vi "SetExposure.vi"(8 "error in (no error)":errorcluster, 10 "Exposure":dbl, 11 "CameraSession  in":refnum<class "CS250-CameraHardwareClass.lvclass">) -> (0 "error out":errorcluster, 1 "Success":bool, 2 "ExposureReadback(Sec)":dbl, 3 "CameraSession out":refnum<class "CS250-CameraHardwareClass.lvclass">)   [LabVIEW 2013, in "CS250-CameraHardwareClass.lvclass"]
uses:
  CS250-CameraHardwareClass.lvclass
  CS250-CameraHardwareClass.lvclass/CS250-CameraHardwareClass.ctl
  Photometrics_CH-250_Cam.lvclass
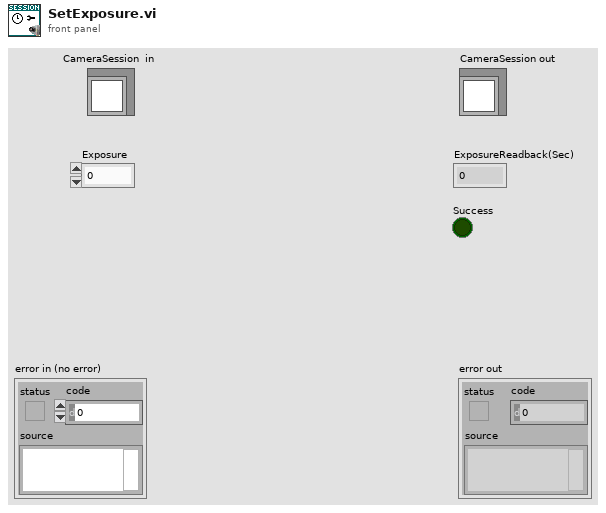
[diagram p1: front panel]
types:
  T1 = typedef "CamCluster.ctl" = cluster{"hcam out":i16, "TempImage":T2, "Pointer":u32, "exp_bytes out":u32, "rgn_array":cluster{"s1":u16, "s2":u16, "sbin":u16, "p1":u16, "p2":u16, "pbin":u16}, "CameraName":string}
  T2 = typedef "IMAQ Image.ctl" = refnum<image>
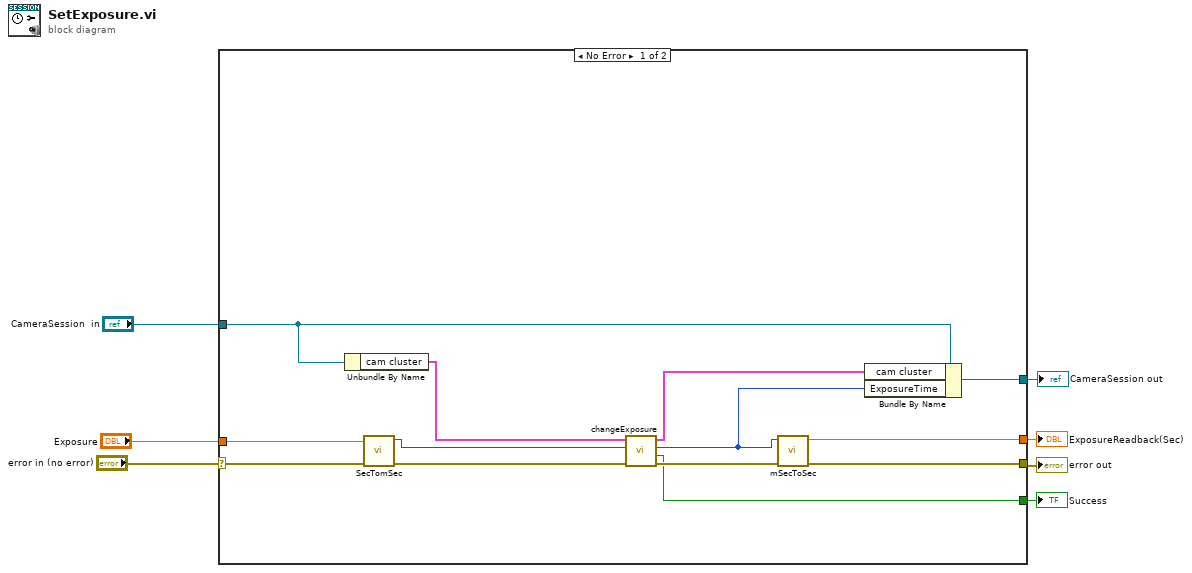
[diagram p0: block diagram]
diagram:
  n1 = case shown="No Error" "error in (no error)" {
    selector: "error in (no error)" -> [w17 w20]
    tunnel: [w16 w20] -> w6
    tunnel: [w13 w19] -> w5
    tunnel: "CameraSession  in" -> [w15 w19]
    tunnel: "Exposure" -> [w12 _]
    tunnel: [w11 _] -> w3
    tunnel: [w9 _] -> w2
    frame No Error {
      n2 = Unbundle By Name(w15) -> ("cam cluster"=w18:T1)
      n3 = call "SecTomSec.vi"("Sec"=w12) -> ("mSec"=w10:u32)  [unwired: 10 in]
      n4 = call "changeExposure.vi"("error in (no error)"=w17, "exposure_time (ms)"=w10, "cam cluster out in"=w18) -> ("error out"=w16:errorcluster, "Success"=w9:bool, "exposureReadback (ms)"=w8:u32, "cam cluster out out"=w14:T1)  [unwired: 5 in]
      n5 = call "mSecToSec.vi"("mSec"=w8) -> ("Sec"=w11:dbl)  [unwired: 10 in]
      n6 = Bundle By Name(cluster=w15, "cam cluster"=w14, "ExposureTime"=w8) -> (w13:refnum<class "CS250-CameraHardwareClass.lvclass">)
    }
    frame Error {
    }
  }
  "error out" <- w6
  "CameraSession out" <- w5
  "ExposureReadback(Sec)" <- w3
  "Success" <- w2
